vi "Build All.vi"(6 "error in":errorcluster, 8 "TargetItem in":refnum<vi>, 9 "Project in":refnum<vi>) -> (0 "error out":errorcluster, 1 "Generated files":path[][](array[path]), 2 "TargetItem out":refnum<vi>, 3 "Project out":refnum<vi>)   [LabVIEW 2011, in "Design Server.lvlib"]
uses:
  Design Server.lvlib
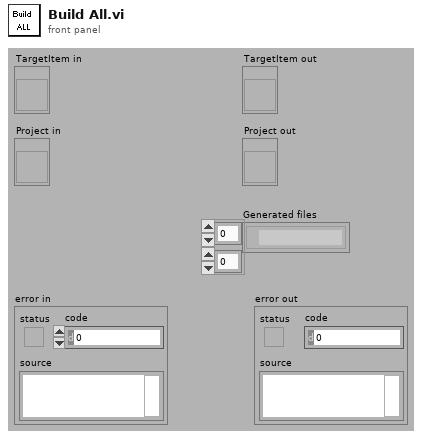
[diagram p1: front panel]
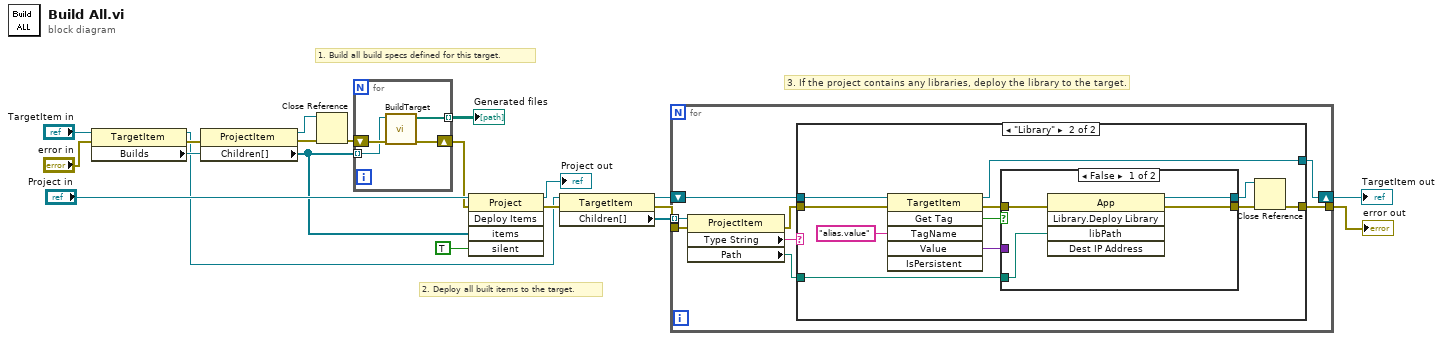
[diagram p0: block diagram]
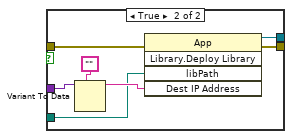
[diagram p3: hidden frame]
diagram:
  # "3. If the project contains any libraries, deploy the library to the target."
  # "2. Deploy all built items to the target."
  # "1. Build all build specs defined for this target."
  n1 = property class="TargetItem"(reference="TargetItem in", error in="error in") -> (reference out=w4:refnum<vi>, error out=w6:errorcluster, "Builds"=w13:refnum<vi>)
  n2 = property class="ProjectItem"(reference=w13, error in=w6) -> (reference out=w2:refnum<vi>, error out=w3:errorcluster, "Children[]"=w8:refnum<vi>[])
  n3 = Close Reference(reference=w2, error in (no error)=w3) -> (error out=w1:errorcluster)
  n4 = for {
    tunnel: w8 -> [w23] mode=indexing
    tunnel: [w22] -> w19 mode=indexing
    shift-right: [w21] -> w7
    shift-left: w1 -> [w24]
    n5 = call <vilib>:"BuildTarget.vi"("error in (no error)"=w24, "BuildItem ref"=w23) -> ("error out"=w21:errorcluster, "Generated files"=w22:path[])  [unwired: 8 out]
  }
  "Generated files" <- w19
  n6 = invoke class="Project" method="Deploy Items"(reference="Project in", error in=w7, "items"=w8, "silent"=TRUE ("Silent")) -> (reference out=→"Project out":refnum<vi>, error out=w9:errorcluster)  [unwired: 1 in, 3 out]
  n7 = property class="TargetItem"(reference=w4, error in=w9) -> (reference out=w18:refnum<vi>, error out=w12:errorcluster, "Children[]"=w11:refnum<vi>[])
  n8 = for {
    tunnel: w11 -> [w32] mode=indexing
    tunnel: w12 -> [w26]
    shift-right: [w29] -> w14
    shift-left: w18 -> [w28]
    tunnel: [w27] -> w20
    n9 = property class="ProjectItem"(reference=w32, error in=w26) -> (error out=w30:errorcluster, "Type String"=w31:string, "Path"=w25:path)  [unwired: 1 out]
    n10 = case shown="\"Library\"" w31 {
      tunnel: w30 -> [w33 w45]
      tunnel: w28 -> [w34 w40]
      tunnel: [w34 w43] -> w29
      tunnel: [w33 w37] -> w27
      tunnel: w25 -> [_ w38]
      frame "", Default {
      }
      frame "Library" {
        n11 = invoke class="TargetItem" method="Get Tag"(reference=w40, error in=w45, "TagName"="alias.value" ("name or relative path")) -> (reference out=w43:refnum<vi>, error out=w39:errorcluster, "GetTag"=w41:bool, "Value"=w42:variant)  [unwired: 3 in, 2 out]
        n12 = case shown="False" w41 {
          tunnel: w42 -> [_ w55]
          tunnel: w39 -> [w49 w53]
          tunnel: [w48 w54] -> w36
          tunnel: w38 -> [w47 w51]
          tunnel: [w46 w50] -> w35
          frame False {
            n13 = invoke class="App" method="Library.Deploy Library"(error in=w49, "libPath"=w47) -> (reference out=w46:refnum<vi>, error out=w48:errorcluster)  [unwired: 3 in, 3 out]
          }
          frame True {
            n14 = Variant To Data(type="" ("data"), Variant=w55) -> (data=w52:string)  [unwired: 1 in, 1 out]
            n15 = invoke class="App" method="Library.Deploy Library"(error in=w53, "libPath"=w51, "Dest IP Address"=w52) -> (reference out=w50:refnum<vi>, error out=w54:errorcluster)  [unwired: 2 in, 3 out]
          }
        }
        n16 = Close Reference(reference=w35, error in (no error)=w36) -> (error out=w37:errorcluster)
      }
    }
  }
  "error out" <- w20
  "TargetItem out" <- w14
